vi "Check Connection.vi"(8 "error in (no error)":errorcluster) -> (0 "error out":errorcluster, 1 "Connected?":bool, 3 "Log Entry":string)   [LabVIEW 2014]
uses:
  Globals/Global - pR netw comm.vi
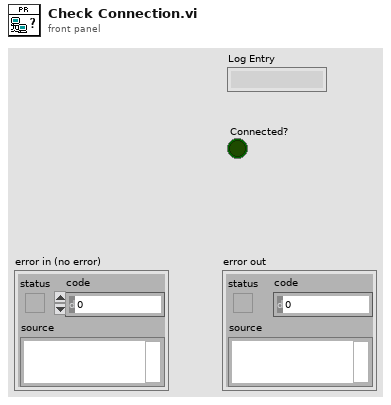
[diagram p1: front panel]
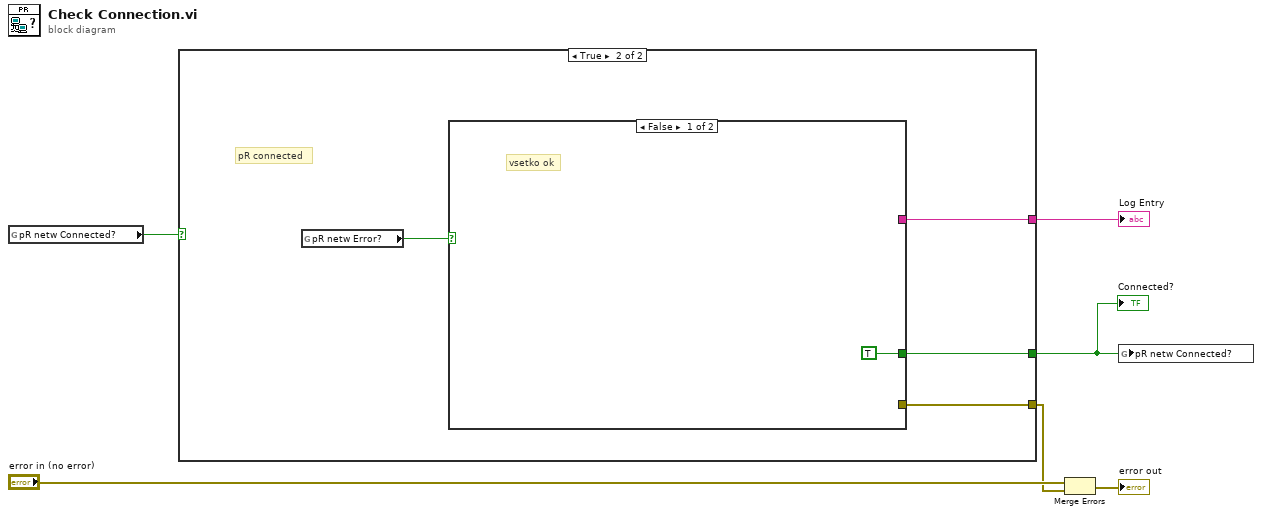
[diagram p0: block diagram]
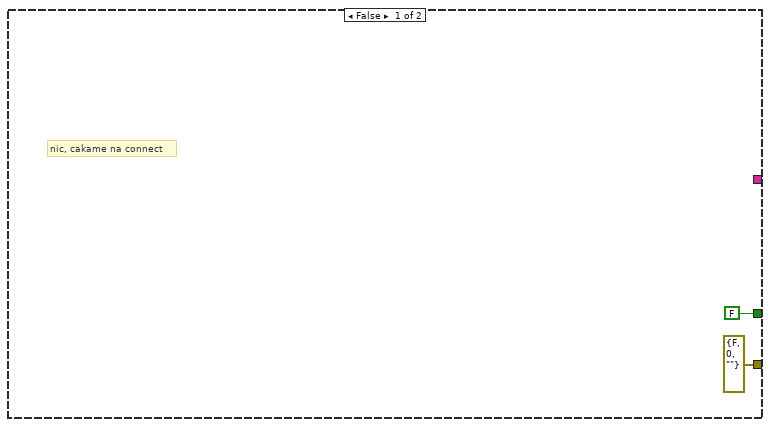
[diagram p2: hidden frame]
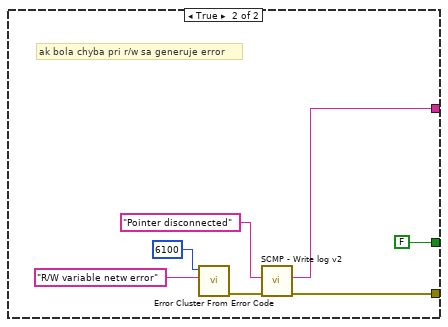
[diagram p3: hidden frame]
diagram:
  n1 = global read "Global - pR netw comm.vi" "pR netw Connected?"() -> (w6:bool)
  n2 = case shown="True" w6 {
    tunnel: [FALSE w11] -> w3
    tunnel: [errorcluster {"status"=FALSE, "code"=0, "source"=""} ("error out") w10] -> w1
    tunnel: [_ w9] -> w2
    frame False {
      # "nic, cakame na connect"
    }
    frame True {
      # "pR connected"
      n3 = global read "Global - pR netw comm.vi" "pR netw Error?"() -> (w12:bool)
      n4 = case shown="False" w12 {
        tunnel: [TRUE FALSE] -> w11
        tunnel: [_ w15] -> w10
        tunnel: [_ w14] -> w9
        frame False {
          # "vsetko ok"
        }
        frame True {
          # "ak bola chyba pri r/w sa generuje error"
          n5 = call <vilib>:"Error Cluster From Error Code.vi"("error message (\"\")"="R/W variable netw error" ("error message (\"\")"), "error code (0)"=6100) -> ("error out"=w18:errorcluster)  [unwired: 7 in]
          n6 = call "SCMP - Write log v2.vi"("Error to log"=w18, "data"="Pointer disconnected") -> ("error out"=w15:errorcluster, "Last Log Entry"=w14:string)  [unwired: 7 in, 1 out]
        }
      }
    }
  }
  "Connected?" <- w3
  "Log Entry" <- w2
  n7 = Merge Errors("error in (no error)", w1) -> (→"error out":errorcluster)
  n8 = global write "Global - pR netw comm.vi" "pR netw Connected?"(w3) -> ()
